vi "Sensors.vi"() -> ()   [LabVIEW 2015]
panel:
  out "Reset Drive Encoders":bool
  out "Limit Switch for Arm Down":bool
  out "Limit Switch for Arm Up":bool
  out "Control on X":dbl
  out "Control on Y":dbl
  out "Motor Output Elbow":dbl
  out "Motor Output Shoulder":dbl
  out "Arm Enabled":bool
  out "Desired angle at 1":dbl
  out "Desired angle at S":dbl
  out "Right Drive v":dbl
  out "Right Drive d":dbl
  out "Shooter Speed":dbl
  out "Limit Switch for Intake":bool
  out "Accelerometer":dbl
  out "Encoder For Arm Shoulder":dbl
  out "Encoder For Arm Joint":dbl
  out "Chassis Gyro":dbl
  out "Left Drive v":dbl
  out "Left Drive d":dbl
  out "Diff Ultrasonic":dbl
  out "Lidar":dbl
  out "Maxsonar":dbl
  out "Infrared":dbl
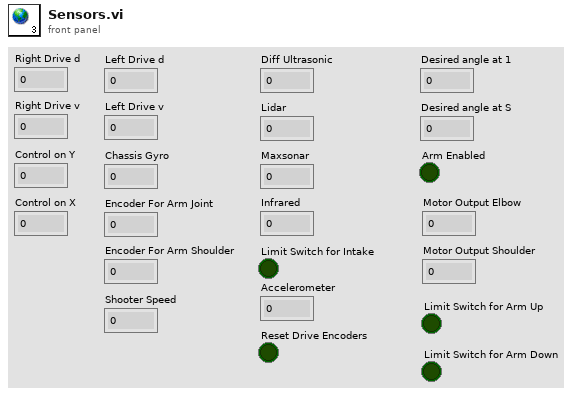
[diagram p1: front panel]
diagram:
